vi "comm flush flags.vi"(1 "flush flags cluster":T1) -> (0 "Flush Flags":u32 format="%.0x")   [LabVIEW 2017, in "lvserial.lvlib"]
uses:
  lvserial.lvlib
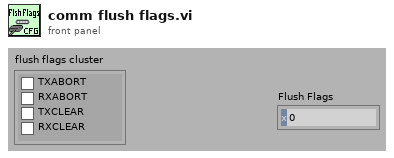
[diagram p1: front panel]
types:
  T1 = cluster{"TXABORT":bool, "RXABORT":bool, "TXCLEAR":bool, "RXCLEAR":bool}
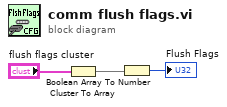
[diagram p0: block diagram]
diagram:
  n1 = Cluster To Array(cluster="flush flags cluster") -> (array=w1:bool[])
  n2 = Boolean Array To Number(Boolean array=w1) -> (number=→"Flush Flags":u32)
